vi "Delta_RH_v2.vi"() -> ()   [LabVIEW 2019]
uses:
  <vilib>/Analysis/baseanly.llb/Mean (DBL).vi
  DeltaRamp_globals.vi
  B_Globals.vi
  Global 2.vi
  <vilib>/Analysis/NI_AALBase.lvlib
panel:
  out "B_set [T]":dbl
  in  "Reading Delay [ms]":i32=100 min=5
  in  "RW Delay":i32=50
  out "Exec Time [ms]":u32
  out "read buffer":string
  in  "B/T":bool
  in  "Smart Avs":bool=TRUE
  in  "Points":dbl=1.0
  out "PpP":dbl
  in  "Combo Box":string(combo)
  in  "Save":bool
  in  "Abort Delta":bool
  out "B [T]":dbl=0.49837
  in  "Arm":bool
  in  "Measure":bool
  in  "Comp":dbl=10.0
  in  "Delay":dbl=0.002
  in  "I_Max":dbl=0.00055
  out "T":cluster{"X":dbl[], "Y":dbl[]}[](graph)=[{"X"=[0.48596000000030654, 0.48632999999976745, 0.4888800000004717, 0.4914299999991856, 0.49799999999988437, 0.49837000000048626, 0.49799999999964834, 0.49764000000059827, 0.4972699999998548, 0.49799999999964706, 0.4976400000005962, 0.4979999999996451, 0.49764000000114167, 0.4987299999995217, 0.49837000000048276, 0.4979999999996453, 0.49764000000060443, 0.4980000000000499, 0.4983700000004744, 0.4979999999996602, 0.4983700000001006, 0.4979999999996734, 0.49764000000018094, 0.4979999999996305, 0.4976400000006558, 0.4979999999996311, 0.4976399999998779, 0.49799999999967304, 0.4983699999999628, 0.49799999999964784, 0.49764000000002906, 0.4983699999999084, 0.49799999999967276, 0.498370000000109, 0.4979999999996426, 0.4983700000001016, 0.4979999999996246, 0.4983700000001098, 0.4979999999996428, 0.4976400000006453], "Y"=[nan, nan, nan, nan, nan, nan, nan, nan, nan, nan, nan, nan, nan, nan, nan, nan, nan, nan, nan, nan, nan, nan, nan, nan, nan, nan, nan, nan, nan, nan, nan, nan, nan, nan, nan, nan, nan, nan, nan, nan]}] caption="XY Graph"
  in  "Reset":bool
  out "Spl T [K]":dbl=6.1992
  out "R [Ohm]":dbl=nan
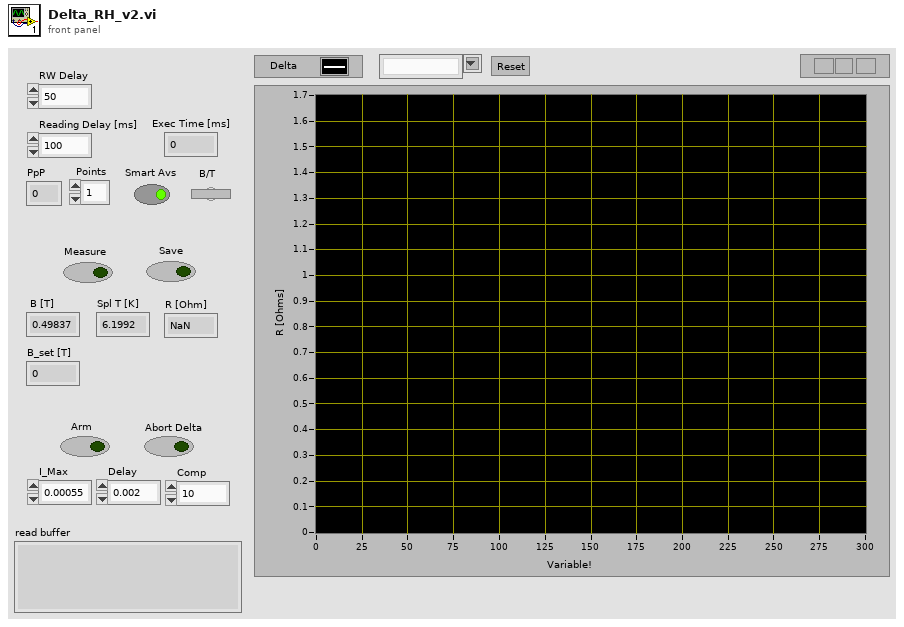
[diagram p1: front panel]
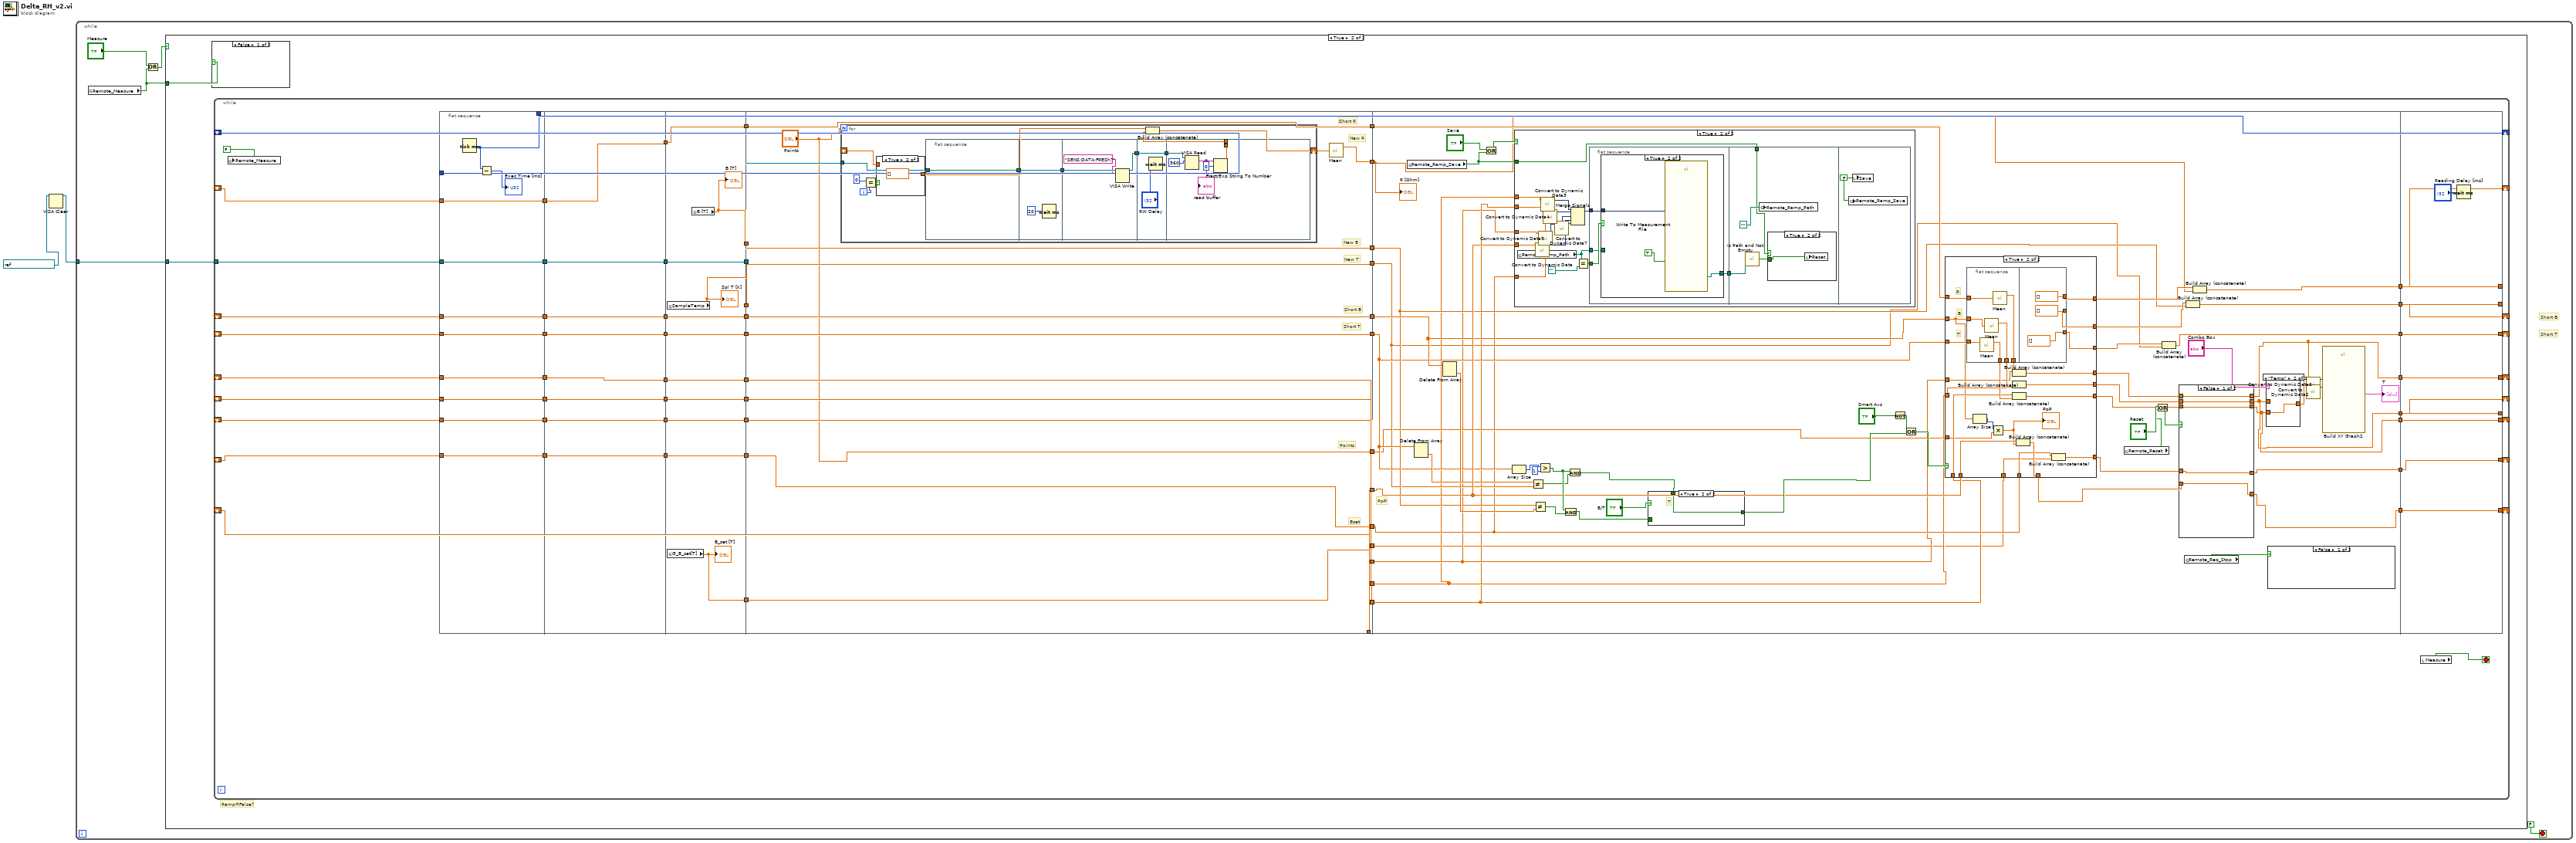
[diagram p0: block diagram]
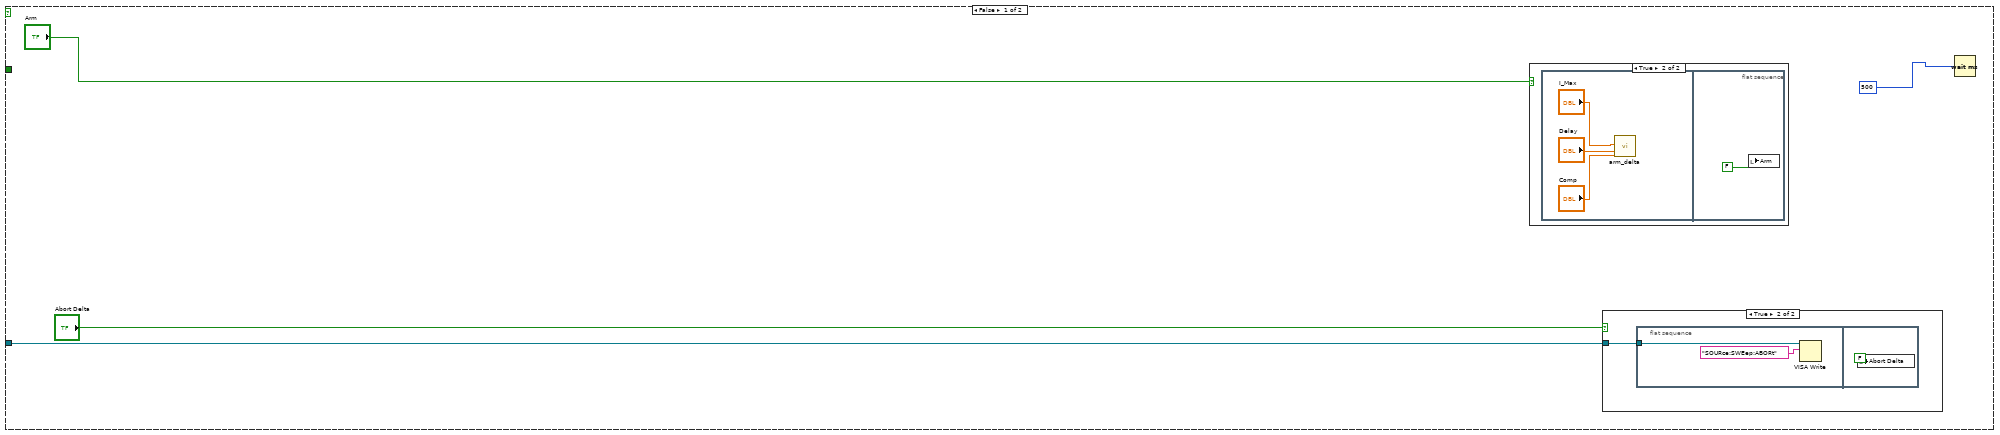
[diagram p2: hidden frame]
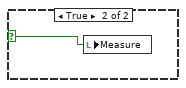
[diagram p5: hidden frame]
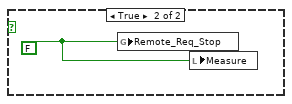
[diagram p8: hidden frame]
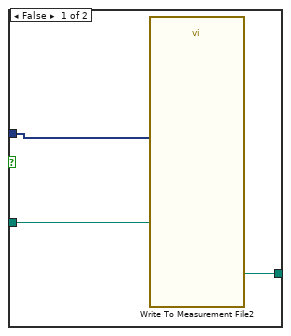
[diagram p12: hidden frame]
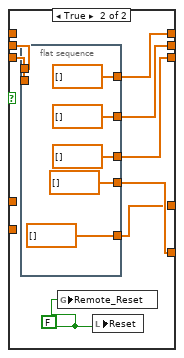
[diagram p14: hidden frame]
diagram:
  n1 = VISA Clear(VISA resource name=refnum<visa-resource-name> "GPIB1::20::INSTR" ("Keithley")) -> (VISA resource name out=w2:refnum<visa-resource-name>)  [unwired: 1 in, 1 out]
  n2 = while {
    tunnel: w2 -> [w6]
    stop <- FALSE stop-if-true
    # "Short T"
    # "Short B"
    n3 = global read "DeltaRamp_globals.vi" "Remote_Measure"() -> (w3:bool)
    n4 = Or(x="Measure", y=w3) -> (x .or. y?=w5:bool)
    n5 = case shown="True" w5 {
      tunnel: w6 -> [w9 w21]
      tunnel: w3 -> [_ w20]
      frame False {
        n6 = case shown="True" "Arm" {
          frame False {
          }
          frame True {
            n7 = flat-sequence {
              frame #0 {
                n8 = call "arm_delta.vi"("Compliance [V]"="Comp", "DELAY [sec]"="Delay", "I-HIGH [A]"="I_Max") -> ()  [unwired: 9 in]
              }
              frame #1 {
                n9 = local write "Arm"(FALSE) -> ()
              }
            }
          }
        }
        n10 = case shown="True" "Abort Delta" {
          tunnel: w9 -> [_ w12]
          frame False {
          }
          frame True {
            n11 = flat-sequence {
              tunnel: w12 -> [w14]
              frame #0 {
                n12 = VISA Write(VISA resource name=w14, write buffer="SOURce:SWEep:ABORt") -> ()  [unwired: 1 in, 3 out]
              }
              frame #1 {
                n13 = local write "Abort Delta"(FALSE) -> ()
              }
            }
          }
        }
        n14 = Wait (ms)(milliseconds to wait=500) -> ()  [unwired: 1 out]
      }
      frame True {
        # "Ramp=False?"
        n15 = case shown="False" w20 {
          selector: w20 -> [_ w22]
          frame False {
          }
          frame True {
            n16 = local write "Measure"(w22) -> ()
          }
        }
        n17 = while {
          shift-right: [w42] -> _
          shift-left: _ -> [w49]
          shift-right: [w61] -> _
          shift-left: _ -> [w66]
          tunnel: w21 -> [w85]
          shift-right: [w59] -> _
          shift-left: _ -> [w72]
          shift-right: [w41] -> _
          shift-left: _ -> [w53]
          shift-right: [w43] -> _
          shift-left: _ -> [w58]
          shift-right: [w60] -> _
          shift-left: _ -> [w76]
          shift-right: [w86] -> _
          shift-left: _ -> [w87]
          shift-right: [w89] -> _
          shift-left: _ -> [w90]
          shift-right: [w25] -> _
          shift-left: _ -> [w30]
          stop <- w32 stop-if-true
          n18 = global write "DeltaRamp_globals.vi" "Remote_Measure"(FALSE) -> ()
          n19 = flat-sequence {
            tunnel: w90 -> [w102]
            tunnel: [w100] -> w89
            tunnel: w85 -> [w99]
            tunnel: [w99] -> w82
            tunnel: w76 -> [w98]
            tunnel: [w98] -> w75
            tunnel: w72 -> [w97]
            tunnel: [w97] -> w69
            tunnel: w66 -> [w96]
            tunnel: [w96] -> w64
            tunnel: w58 -> [w95]
            tunnel: [w95] -> w55
            tunnel: [w94] -> w54
            tunnel: w53 -> [w94]
            tunnel: [w93] -> w50
            tunnel: w49 -> [w93]
            tunnel: [w92] -> w31
            tunnel: w30 -> [w92]
            tunnel: [w110] -> w83
            tunnel: w82 -> [w110]
            tunnel: w75 -> [w109]
            tunnel: [w109] -> w74
            tunnel: [w108] -> w70
            tunnel: w69 -> [w108]
            tunnel: [w107] -> w65
            tunnel: w64 -> [w107]
            tunnel: [w106] -> w56
            tunnel: w55 -> [w106]
            tunnel: w54 -> [w105]
            tunnel: [w105] -> w51
            tunnel: w50 -> [w104]
            tunnel: [w104] -> w47
            tunnel: w31 -> [w103]
            tunnel: [w103] -> w28
            tunnel: [w121] -> w84
            tunnel: w83 -> [w121]
            tunnel: [w120] -> w80
            tunnel: [w119] -> w78
            tunnel: w74 -> [w118]
            tunnel: [w118] -> w73
            tunnel: [w117] -> w71
            tunnel: w70 -> [w117]
            tunnel: w65 -> [w116]
            tunnel: [w116] -> w63
            tunnel: [w115] -> w57
            tunnel: w56 -> [w115]
            tunnel: [w114] -> w52
            tunnel: w51 -> [w114]
            tunnel: [w113] -> w48
            tunnel: w47 -> [w113]
            tunnel: [w112] -> w29
            tunnel: w28 -> [w112]
            tunnel: [w111] -> w24
            tunnel: [w135] -> w88
            tunnel: w87 -> [w135]
            tunnel: w84 -> [w134]
            tunnel: [w133] -> w81
            tunnel: w80 -> [w132]
            tunnel: [w132] -> w79
            tunnel: w78 -> [w131]
            tunnel: [w131] -> w77
            tunnel: w73 -> [w130]
            tunnel: w71 -> [w129]
            tunnel: [w130] -> w68
            tunnel: [w129] -> w67
            tunnel: w63 -> [w128]
            tunnel: [w128] -> w62
            tunnel: w57 -> [w127]
            tunnel: w52 -> [w126]
            tunnel: w48 -> [w125]
            tunnel: [w127] -> w46
            tunnel: [w126] -> w45
            tunnel: [w125] -> w44
            tunnel: ["Points"] -> w40
            tunnel: w29 -> [w123]
            tunnel: [w123] -> w27
            tunnel: w24 -> [w122]
            tunnel: [w122] -> w23
            tunnel: w88 -> [w192]
            tunnel: w81 -> [w184]
            tunnel: w79 -> [w183]
            tunnel: w77 -> [w179]
            tunnel: w68 -> [w188]
            tunnel: w67 -> [w182]
            tunnel: w62 -> [w187]
            tunnel: w46 -> [w167]
            tunnel: w45 -> [w166]
            tunnel: w44 -> [w165]
            tunnel: w40 -> [w171]
            tunnel: [w172] -> w39
            tunnel: [w185] -> w38
            tunnel: [w181] -> w37
            tunnel: [w180] -> w36
            tunnel: [w178] -> w35
            tunnel: [w174] -> w34
            tunnel: [w173] -> w33
            tunnel: w27 -> [w168]
            tunnel: [w170] -> w26
            tunnel: w23 -> [w164]
            tunnel: [w316] -> w41
            tunnel: [w317] -> w42
            tunnel: [w318] -> w43
            tunnel: [w319] -> w59
            tunnel: [w320] -> w60
            tunnel: [w321] -> w61
            tunnel: [w322] -> w86
            tunnel: w39 -> [w322]
            tunnel: w38 -> [w321]
            tunnel: w37 -> [w320]
            tunnel: w36 -> [w319]
            tunnel: w35 -> [w318]
            tunnel: w34 -> [w317]
            tunnel: w33 -> [w316]
            tunnel: w26 -> [w314]
            tunnel: [w314] -> w25
            frame #0 {
              n20 = Tick Count (ms)() -> (millisecond timer value=w100:u32)
              n21 = Subtract(x=w100, y=w102) -> (x-y=→"Exec Time [ms]":u32)
            }
            frame #1 {
            }
            frame #2 {
              n22 = global read "Global 2.vi" "SampleTemp"() -> (w119:dbl)
              "Spl T [K]" <- w119
              n23 = global read "B_Globals.vi" "G_B_set[T]"() -> (w111:dbl)
              "B_set [T]" <- w111
              n24 = global read "B_Globals.vi" "B [T]"() -> (w120:dbl)
              "B [T]" <- w120
            }
            frame #3 {
              # "Bset"
              # "Points"
              # "Short R"
              # "New T"
              # "New B"
              # "Short T"
              # "Short B"
              # "New R"
              n25 = for {
                N: "Points" -> [_]
                tunnel: w134 -> [w148]
                shift-right: [w147] -> w136
                shift-left: _ -> [w139]
                i -> [w141]
                n26 = Equal?(x=0, y=w141) -> (x = y?=w143:bool)
                n27 = case shown="True" w143 {
                  tunnel: [w149 dbl[] [] ("Numeric")] -> w140
                  tunnel: w139 -> [w149 _]
                  frame False {
                  }
                  frame True {
                  }
                }
                n28 = flat-sequence {
                  tunnel: w148 -> [w151]
                  tunnel: [w151] -> w138
                  tunnel: w138 -> [w153]
                  tunnel: [w153] -> w137
                  tunnel: [w155] -> w144
                  tunnel: w137 -> [w156]
                  tunnel: [w157] -> w145
                  tunnel: w144 -> [w157]
                  tunnel: w145 -> [w160]
                  tunnel: [w161] -> w146
                  tunnel: [w161] -> _
                  frame #0 {
                  }
                  frame #1 {
                    n29 = Wait (ms)(milliseconds to wait=20) -> ()  [unwired: 1 out]
                  }
                  frame #2 {
                    n30 = VISA Write(VISA resource name=w156, write buffer="SENS:DATA:FRESh?" ("write buffer 2")) -> (VISA resource name out=w155:refnum<visa-resource-name>)  [unwired: 1 in, 2 out]
                  }
                  frame #3 {
                    n31 = Wait (ms)(milliseconds to wait="RW Delay") -> ()  [unwired: 1 out]
                  }
                  frame #4 {
                    n32 = VISA Read(VISA resource name=w160, byte count=u32 360) -> (read buffer=w159:string)  [unwired: 1 in, 3 out]
                    "read buffer" <- w159
                    n33 = Fract/Exp String To Number(string=w159, offset=0) -> (number=w161:dbl)  [unwired: 3 out]
                  }
                }
                n34 = Build Array (concatenate)(w140, w146) -> (w147:dbl[])
              }
              n35 = call-poly <vilib>:"Mean.vi"("X"=w136) -> ("mean"=w133:dbl)  [unwired: 1 out]
            }
            frame #4 {
              # "PpP"
              n36 = global read "DeltaRamp_globals.vi" "Remote_Ramp_Save"() -> (w204:bool)
              n37 = Delete From Array(array=w182) -> (deleted portion=w190:dbl)  [unwired: 2 in, 1 out]
              n38 = Delete From Array(array=w188) -> (deleted portion=w189:dbl)  [unwired: 2 in, 1 out]
              n39 = Or(x="Save", y=w204) -> (x .or. y?=w199:bool)
              n40 = Array Size(array=w182) -> (size(s)=w209:i32)
              n41 = case shown="True" w199 {
                tunnel: w204 -> [_ w271]
                tunnel: w192 -> [_ w270]
                tunnel: w168 -> [_ w265]
                tunnel: w167 -> [_ w268]
                tunnel: w166 -> [_ w267]
                tunnel: w165 -> [_ w266]
                frame False {
                }
                frame True {
                  n42 = global read "DeltaRamp_globals.vi" "Remote_Ramp_Path"() -> (w273:path)
                  n43 = call "Convert to Dynamic Data"("Array"=w270) -> ("Dynamic Data Type"=w269:dynamicdata)  [unwired: 3 in]
                  n44 = call "Convert to Dynamic Data5"("Array"=w268) -> ("Dynamic Data Type"=w276:dynamicdata)  [unwired: 3 in]
                  n45 = call "Convert to Dynamic Data3"("Array"=w267) -> ("Dynamic Data Type"=w278:dynamicdata)  [unwired: 3 in]
                  n46 = call "Convert to Dynamic Data4"("Array"=w266) -> ("Dynamic Data Type"=w277:dynamicdata)  [unwired: 3 in]
                  n47 = call "Convert to Dynamic Data7"("Array"=w265) -> ("Dynamic Data Type"=w264:dynamicdata)  [unwired: 3 in]
                  n48 = Merge Signals(w278, w277, w276, w269, w264) -> (w279:dynamicdata)
                  n49 = Equal?(x=w273, y=path "") -> (x = y?=w274:bool)
                  n50 = flat-sequence {
                    tunnel: w279 -> [w283]
                    tunnel: w274 -> [w282]
                    tunnel: w273 -> [w281]
                    tunnel: [w280] -> w272
                    tunnel: w272 -> [w292]
                    tunnel: w271 -> [w291]
                    frame #0 {
                      n51 = case shown="True" w282 {
                        tunnel: w283 -> [w286 w288]
                        tunnel: w281 -> [w285 _]
                        tunnel: [w284 w287] -> w280
                        frame False {
                          n52 = call "Write To Measurement File2"("Signals"=w286, "Filename"=w285) -> ("Filename Out"=w284:path)  [unwired: 15 in, 2 out]
                        }
                        frame True {
                          n53 = call "Write To Measurement File"("Signals"=w288, "Reset"=TRUE) -> ("Filename Out"=w287:path)  [unwired: 15 in, 2 out]
                        }
                      }
                    }
                    frame #1 {
                      n54 = call <vilib>:"Is Path and Not Empty.vi"("path"=w292) -> ("Is Path and Not Empty?"=w290:bool)  [unwired: 4 in]
                      n55 = global write "DeltaRamp_globals.vi" "Remote_Ramp_Path"(path "") -> ()
                      n56 = case shown="True" w291 {
                        tunnel: w290 -> [_ w294]
                        frame False {
                        }
                        frame True {
                          n57 = local write "Reset"(w294) -> ()
                        }
                      }
                    }
                    frame #2 {
                      w295 = FALSE
                      n58 = global write "DeltaRamp_globals.vi" "Remote_Ramp_Save"(w295) -> ()
                      n59 = local write "Save"(w295) -> ()
                    }
                  }
                }
              }
              n60 = Not Equal?(x=w190, y=w179) -> (x != y?=w210:bool)
              n61 = Not Equal?(x=w183, y=w189) -> (x != y?=w213:bool)
              n62 = Greater?(x=w209, y=1) -> (0:w212:bool)
              n63 = And(x=w212, y=w213) -> (x .and. y?=w214:bool)
              n64 = And(x=w212, y=w210) -> (x .and. y?=w215:bool)
              n65 = case shown="True" "B/T" {
                tunnel: w214 -> [w219 _]
                tunnel: w215 -> [_ w220]
                tunnel: [w219 w220] -> w216
                frame False {
                  # "B"
                }
                frame True {
                  # "T"
                }
              }
              n66 = Not(x="Smart Avs") -> (.not. x?=w206:bool)
              n67 = Or(x=w206, y=w216) -> (x .or. y?=w207:bool)
              n68 = case shown="True" w207 {
                tunnel: [w228 w252] -> w218
                tunnel: [w226 w251] -> w186
                tunnel: [w227 w238] -> w217
                tunnel: [w223 w249] -> w195
                tunnel: [w225 w248] -> w196
                tunnel: [w224 w246] -> w197
                tunnel: [w229 w244] -> w191
                tunnel: w192 -> [w229 w243]
                tunnel: w188 -> [w228 w234]
                tunnel: w182 -> [w227 w239]
                tunnel: w187 -> [w226 w240]
                tunnel: w167 -> [w225 w237]
                tunnel: w166 -> [w223 w236]
                tunnel: w165 -> [w224 w235]
                tunnel: w171 -> [_ w233]
                tunnel: w168 -> [w222 w232]
                tunnel: [w222 w231] -> w169
                tunnel: w164 -> [_ w230]
                frame False {
                }
                frame True {
                  # "T"
                  # "B"
                  # "R"
                  n69 = flat-sequence {
                    tunnel: [w257] -> w250
                    tunnel: [w256] -> w245
                    tunnel: [w258] -> w247
                    tunnel: w240 -> [w255]
                    tunnel: w234 -> [w254]
                    tunnel: w239 -> [w253]
                    tunnel: [dbl[] []] -> w238
                    tunnel: [dbl[] []] -> w252
                    tunnel: [dbl[] []] -> w251
                    frame #0 {
                      n70 = call-poly <vilib>:"Mean.vi"("X"=w253) -> ("mean"=w258:dbl)  [unwired: 1 out]
                      n71 = call-poly <vilib>:"Mean.vi"("X"=w254) -> ("mean"=w257:dbl)  [unwired: 1 out]
                      n72 = call-poly <vilib>:"Mean.vi"("X"=w255) -> ("mean"=w256:dbl)  [unwired: 1 out]
                    }
                    frame #1 {
                    }
                  }
                  n73 = Array Size(array=w234) -> (size(s)=w242:i32)
                  n74 = Multiply(x=w242, y=w233) -> (x*y=w241:dbl)
                  "PpP" <- w241
                  n75 = Build Array (concatenate)(w237, w245) -> (w248:dbl[])
                  n76 = Build Array (concatenate)(w236, w250) -> (w249:dbl[])
                  n77 = Build Array (concatenate)(w235, w247) -> (w246:dbl[])
                  n78 = Build Array (concatenate)(w243, w241) -> (w244:dbl[])
                  n79 = Build Array (concatenate)(w232, w230) -> (w231:dbl[])
                }
              }
              n80 = global read "DeltaRamp_globals.vi" "Remote_Reset"() -> (w200:bool)
              n81 = Or(x="Reset", y=w200) -> (x .or. y?=w202:bool)
              n82 = Build Array (concatenate)(w217, w179) -> (w180:dbl[])
              n83 = case shown="False" w202 {
                tunnel: w195 -> [w300 w308]
                tunnel: [w300 w307] -> w173
                tunnel: w197 -> [w299 w306]
                tunnel: [w299 w305] -> w174
                tunnel: [w298 w304] -> w178
                tunnel: w196 -> [w298 _]
                tunnel: [w297 w302] -> w172
                tunnel: w191 -> [w297 _]
                tunnel: [w296 w301] -> w170
                tunnel: w169 -> [w296 _]
                frame False {
                }
                frame True {
                  w303 = FALSE
                  n84 = flat-sequence {
                    tunnel: w308 -> [_]
                    tunnel: w306 -> [_]
                    tunnel: [dbl[] []] -> w305
                    tunnel: [dbl[] []] -> w307
                    tunnel: [dbl[] []] -> w304
                    tunnel: [dbl[] [] ("Numeric")] -> w302
                    tunnel: [dbl[] [] ("Numeric")] -> w301
                    frame #0 {
                    }
                  }
                  n85 = global write "DeltaRamp_globals.vi" "Remote_Reset"(w303) -> ()
                  n86 = local write "Reset"(w303) -> ()
                }
              }
              n87 = global read "DeltaRamp_globals.vi" "Remote_Req_Stop"() -> (w203:bool)
              n88 = Build Array (concatenate)(w218, w183) -> (w181:dbl[])
              n89 = Build Array (concatenate)(w186, w184) -> (w185:dbl[])
              n90 = case shown="\"Temp\"" "Combo Box" {
                tunnel: [w262 w263] -> w176
                tunnel: w174 -> [_ w263]
                tunnel: w173 -> [w262 _]
                frame "Field", Default {
                }
                frame "Temp" {
                }
              }
              n91 = case shown="False" w203 {
                frame False {
                }
                frame True {
                  w221 = FALSE
                  n92 = global write "DeltaRamp_globals.vi" "Remote_Req_Stop"(w221) -> ()
                  n93 = local write "Measure"(w221) -> ()
                }
              }
              n94 = call "Convert to Dynamic Data6"("Array"=w176) -> ("Dynamic Data Type"=w175:dynamicdata)  [unwired: 3 in]
              n95 = call "Convert to Dynamic Data2"("Array"=w178) -> ("Dynamic Data Type"=w177:dynamicdata)  [unwired: 3 in]
              n96 = call "Build XY Graph2"("Y Input"=w177, "X Input"=w175) -> ("XY Graph"=→"T":cluster{"X":dbl[], "Y":dbl[]}[])  [unwired: 8 in, 1 out]
              "R [Ohm]" <- w184
            }
            frame #5 {
              n97 = Wait (ms)(milliseconds to wait="Reading Delay [ms]") -> ()  [unwired: 1 out]
            }
          }
          n98 = local read "Measure"() -> (w32:bool)
        }
      }
    }
  }
